vi "DHE_ShareNewExp.vi"(8 "error in (no error)":errorcluster, 10 "UT in":string) -> (0 "error out":errorcluster, 2 "expID":string)   [LabVIEW 2016]
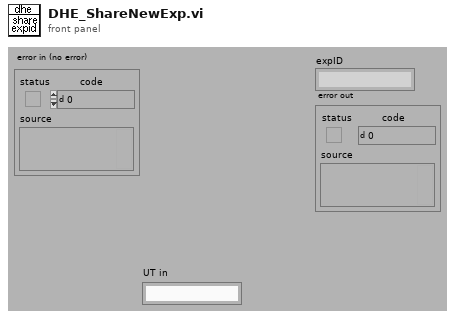
[diagram p1: front panel]
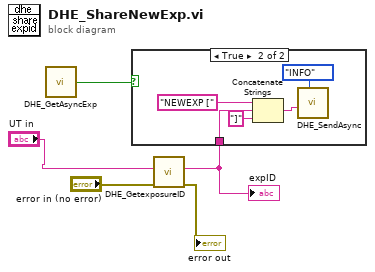
[diagram p0: block diagram]
diagram:
  n1 = call "DHE_GetAsyncExp.vi"() -> ("DHE_asyncexp"=w2:bool)  [unwired: 9 out]
  n2 = call "DHE_GetexposureID.vi"("error in (no error)"="error in (no error)", "UT in"="UT in") -> ("error out"=→"error out":errorcluster, "expID"=w4:string)  [unwired: 8 out]
  "expID" <- w4
  n3 = case shown="True" w2 {
    tunnel: w4 -> [_ w7]
    frame False {
    }
    frame True {
      n4 = Concatenate Strings("NEWEXP [" ("string"), w7, "]" ("string")) -> (w8:string)
      n5 = call "DHE_SendAsync.vi"("type"=enum16{"ERROR", "WARNING", "INFO", "CHANGED"}."INFO", "Message"=w8) -> ()  [unwired: 2 in, 8 out]
    }
  }
